vi "RDS Serial Send Frame.vi"(8 "error in (no error)":errorcluster, 10 "RDS Frame":refnum<class "RDS Serial Frame.lvclass">, 11 "RDS Serial Instrument Actor in":refnum<class "RDS Serial Instrument Actor.lvclass">) -> (0 "error out":errorcluster, 3 "RDS Serial Instrument Actor out":refnum<class "RDS Serial Instrument Actor.lvclass">)   [LabVIEW 2015, in "RDS Abstracts.lvlib" / "RDS Serial Instrument Actor.lvlib" / "RDS Serial Instrument Actor.lvclass"]
uses:
  RDS Serial Instrument Actor.lvclass
  Libraries/RDS Serial Handler/RDS Serial Frame.lvclass
  RDS Serial Instrument Actor.lvclass/RDS Serial Instrument Actor.ctl
  Libraries/RDS Serial Handler/RDS Serial Instrument.lvclass
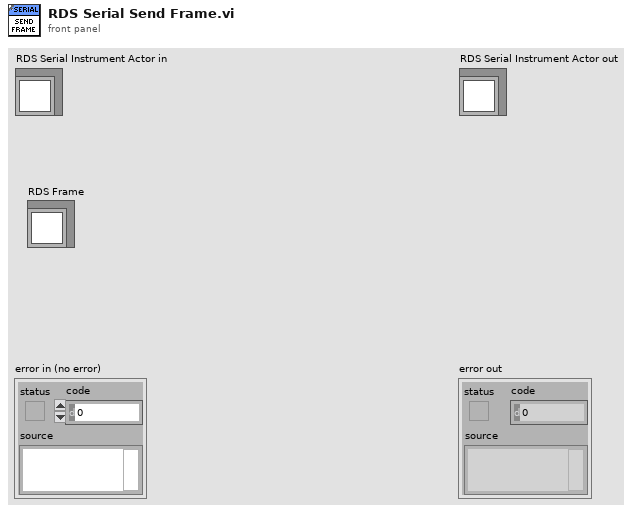
[diagram p1: front panel]
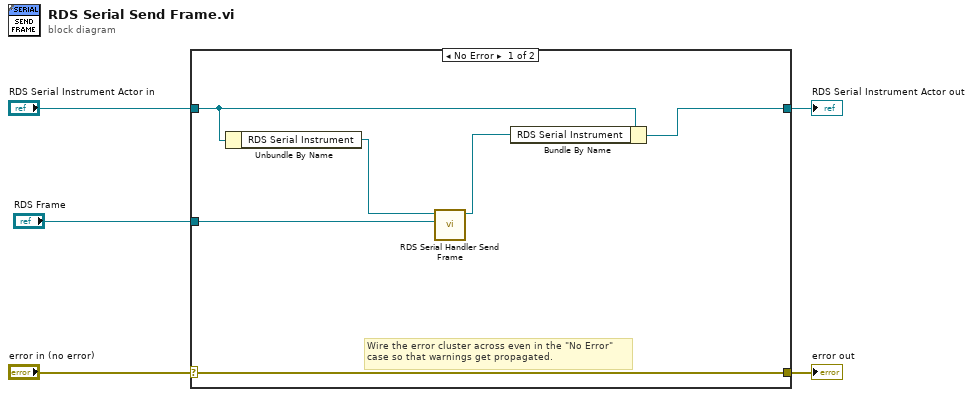
[diagram p0: block diagram]
diagram:
  n1 = case shown="No Error" "error in (no error)" {
    selector: "error in (no error)" -> [w11 w13]
    tunnel: [w11 w13] -> w4
    tunnel: [w6 w12] -> w2
    tunnel: "RDS Serial Instrument Actor in" -> [w7 w12]
    tunnel: "RDS Frame" -> [w10 _]
    frame No Error {
      # "Wire the error cluster across even in the \"No Error\"\ncase so that warnings get propagated."
      n2 = Unbundle By Name(w7) -> ("RDS Serial Instrument"=w9:refnum<class "RDS Serial Instrument.lvclass">)
      n3 = call "RDS Serial Handler Send Frame.vi"("Serial Frame"=w10, "RDS Serial Instrument in"=w9) -> ("RDS Serial Instrument out"=w8:refnum<class "RDS Serial Instrument.lvclass">)  [unwired: 8 in, 1 out]
      n4 = Bundle By Name(cluster=w7, "RDS Serial Instrument"=w8) -> (w6:refnum<class "RDS Serial Instrument Actor.lvclass">)
    }
    frame Error {
    }
  }
  "error out" <- w4
  "RDS Serial Instrument Actor out" <- w2
